vi "Actor Core.vi"(8 "error in":errorcluster, 11 "Example View in":refnum<class "Example View Actor.lvclass">) -> (0 "error out":errorcluster, 3 "Actor out":refnum<class "Actor.lvclass">)   [LabVIEW 2023, in "Example View Actor.lvlib" / "Example View Actor.lvclass"]
doc: "(<B>Filename</B>: Actor Framework.lvlib:Actor.lvclass:Actor Core.vi)\n\nReceives messages to the actor, reacts to them, and initiates any error handling that may shut the actor down.\n\nDescendant classes may override this VI to append parallel tasks for the actor to complete while it handles messages. Overrides use the Call Parent Method node."
uses:
  Example View Actor.lvclass
  <vilib>/ActorFramework/Actor/Actor.lvclass
  View Actor Messages/Generate and Broadcast Event Msg/Generate and Broadcast Event Msg.lvclass
  View Actor/View Actor.lvclass
  Example Events/Boolean Event.lvclass
panel:
  out "Inited At":string
  out "View Name":string
  in  "Boolean":bool
  out "Time":string
  out "Waveform Graph":dbl[](graph)
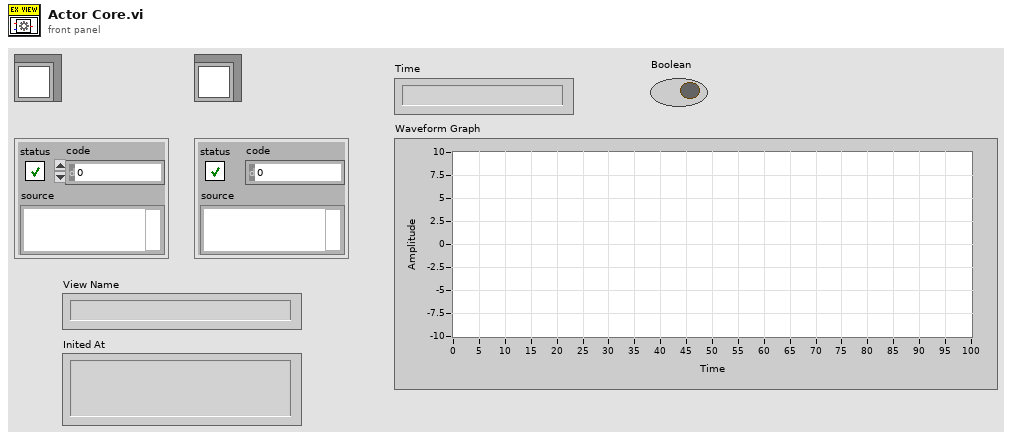
[diagram p1: front panel]
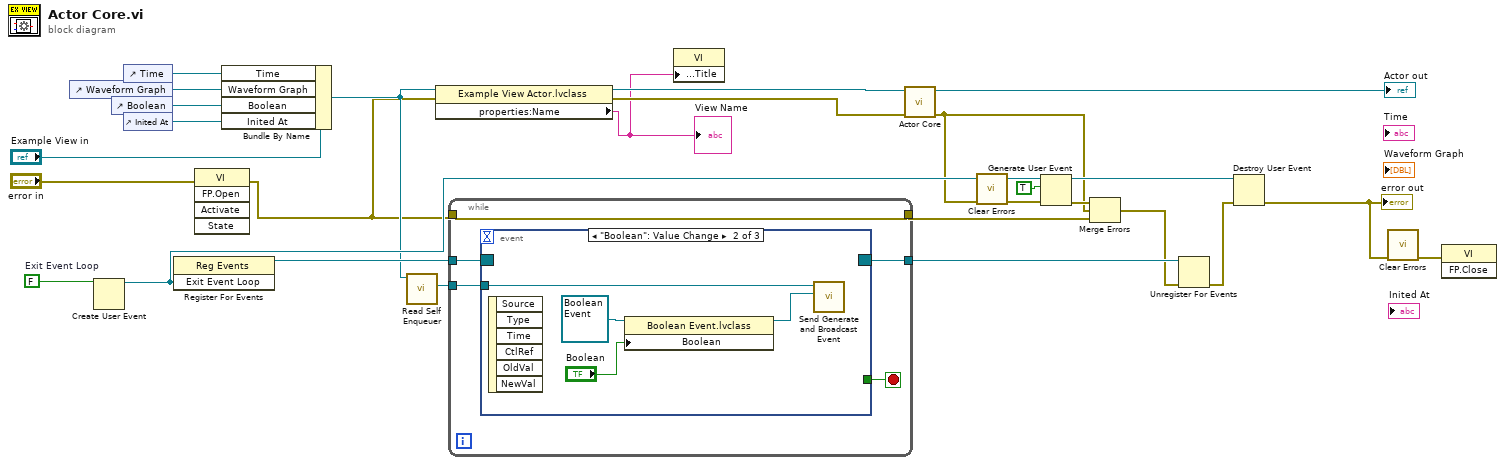
[diagram p0: block diagram]
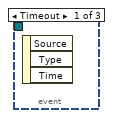
[diagram p2: hidden frame]
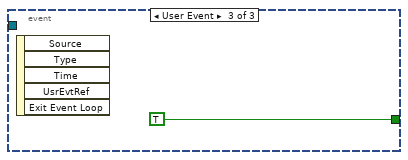
[diagram p3: hidden frame]
diagram:
  w20 = FALSE  # Exit Event Loop
  n1 = control-ref of="Waveform Graph"() -> (w24:refnum<vi>)
  n2 = Create User Event(user event datatype=w20) -> (user event=w17:refnum<user-event>)  [unwired: 1 in, 1 out]
  n3 = control-ref of="Boolean"() -> (w23:refnum<vi>)
  n4 = control-ref of="Time"() -> (w25:refnum<vi>)
  n5 = control-ref of="Inited At"() -> (w1:refnum<vi>)
  n6 = register-events(w17) -> (reference out=w19:refnum<event-registration>)  [unwired: 2 in, 1 out]
  n7 = invoke class="VI" method="FP.Open"(error in="error in") -> (error out=w4:errorcluster)  [unwired: 4 in, 4 out]
  n8 = Bundle By Name(cluster="Example View in", "Time"=w25, "Waveform Graph"=w24, "Boolean"=w23, "Inited At"=w1) -> (w12:refnum<class "Example View Actor.lvclass">)
  n9 = call <vilib>:"Read Self Enqueuer.vi"("Actor"=w12) -> ("Self Enqueuer"=w21:refnum<class "Message Enqueuer.lvclass">)  [unwired: 10 in]
  n10 = property class="Example View Actor.lvclass"(reference=w12, error in=w4) -> (reference out=w5:refnum<class "Example View Actor.lvclass">, error out=w3:errorcluster, "properties:Name"=w2:string)
  "View Name" <- w2
  n11 = while {
    tunnel: w21 -> [w32]
    tunnel: w19 -> [w31]
    tunnel: w4 -> [w30]
    tunnel: [w30] -> w11
    tunnel: [w29] -> w15
    stop <- w28 stop-if-true
    n12 = event shown="[1] \"Boolean\": Value Change" {
      selector: w31 -> [_ _ _]
      dyn-events: [_ _ _] -> w29
      timeout: _ -> [_ _ _]
      tunnel: w32 -> [_ w36 _]
      tunnel: [_ _ TRUE] -> w28
      event Timeout {
        n13 = event-data() -> ()  [unwired: 1 in, 3 out]
      }
      event "Boolean": Value Change {
        n14 = event-data() -> ()  [unwired: 1 in, 6 out]
        n15 = property class="Boolean Event.lvclass"(reference=refnum<class "Boolean Event.lvclass"> refnum ("Example Source.lvlib:Boolean Event.lvclass"), "Boolean"="Boolean") -> (reference out=w33:refnum<class "Boolean Event.lvclass">)  [unwired: 1 in, 1 out]
        n16 = call "Send Generate and Broadcast Event.vi"("Event Data"=w33, "Message Enqueuer in"=w36) -> ()  [unwired: 8 in, 2 out]
      }
      event User Event {
        n17 = event-data() -> ()  [unwired: 1 in, 5 out]
      }
    }
  }
  n18 = property class="VI"("Front Panel.Title"=w2) -> ()  [unwired: 2 in, 2 out]
  n19 = call-parent "Actor Core.vi"("error in"=w3, "Actor in"=w5) -> ("error out"=w7:errorcluster, "Actor out"=→"Actor out":refnum<class "Actor.lvclass">)  [unwired: 8 in]
  n20 = call <vilib>:"Clear Errors.vi"("error in (no error)"=w7) -> ("error out"=w6:errorcluster)  [unwired: 5 in, 1 out]
  n21 = Generate User Event(user event=w17, event data cluster=TRUE ("event data"), error in=w6) -> (user event out=w16:refnum<user-event>, error out=w18:errorcluster)  [unwired: 1 in]
  n22 = Merge Errors(w18, w7, w11) -> (w8:errorcluster)
  n23 = Unregister For Events(event registration refnum=w15, error in=w8) -> (error out=w14:errorcluster)
  n24 = Destroy User Event(user event=w16, error in=w14) -> (error out=w9:errorcluster)
  "error out" <- w9
  n25 = call <vilib>:"Clear Errors.vi"("error in (no error)"=w9) -> ("error out"=w10:errorcluster)  [unwired: 5 in, 1 out]
  n26 = invoke class="VI" method="FP.Close"(error in=w10) -> ()  [unwired: 2 in, 3 out]
